vi "Thread@Suspend__Parameter.vi"(1 "ParamterIn":string) -> (0 "ParamterOut":string)   [LabVIEW 2020]
panel:
  in  "Logic":string(combo)
  in  "Thread":string(combo)="1"
  in  "Confirm":bool
  # "Thread@Suspend $ThreadNo (, $Logic)"
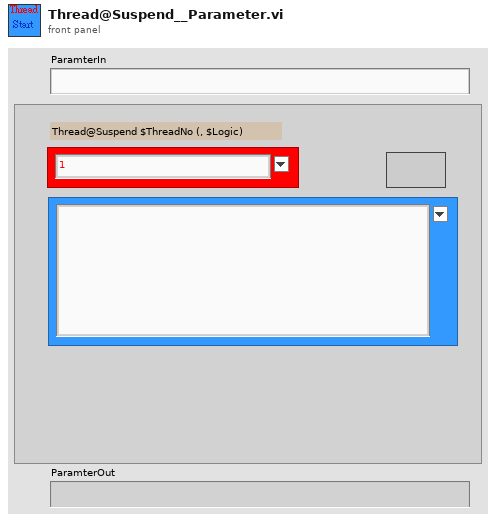
[diagram p1: front panel]
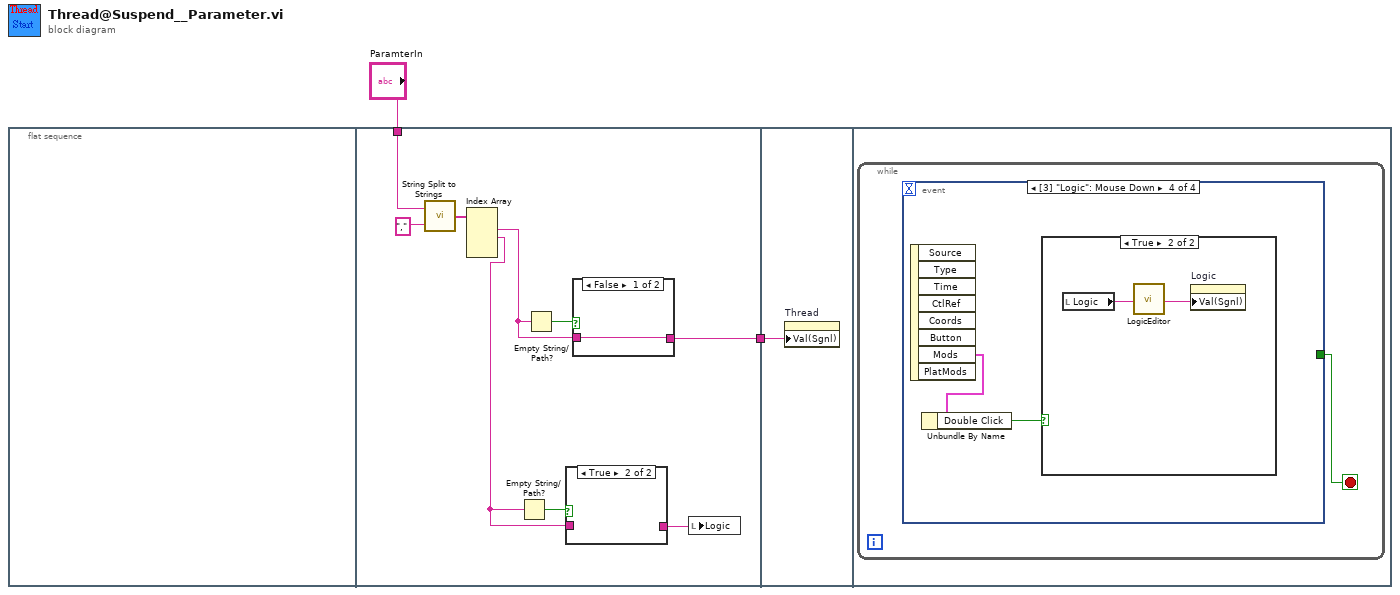
[diagram p0: block diagram]
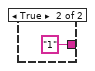
[diagram p3: hidden frame]
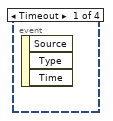
[diagram p4: hidden frame]
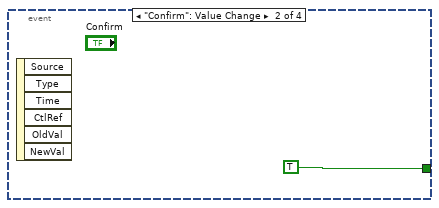
[diagram p5: hidden frame]
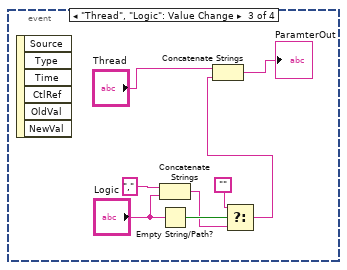
[diagram p6: hidden frame]
diagram:
  n1 = flat-sequence {
    tunnel: "ParamterIn" -> [w9]
    tunnel: [w3] -> w1
    tunnel: w1 -> [w15]
    frame #0 {
    }
    frame #1 {
      n2 = call "String Split to Strings.vi"("search string/char (-)"=",", "String"=w9) -> ("Array"=w11:string[])
      n3 = Index Array(array=w11) -> (element #1=w5:string, element #2=w4:string)  [unwired: 4 in, 2 out]
      n4 = Empty String/Path?(string/path=w4) -> (empty?=w7:bool)
      n5 = Empty String/Path?(string/path=w5) -> (empty?=w8:bool)
      n6 = case shown="True" w7 {
        tunnel: w4 -> [w12 _]
        tunnel: [w12 _] -> w6
        frame False {
        }
        frame True {
        }
      }
      n7 = case shown="False" w8 {
        tunnel: w5 -> [w13 _]
        tunnel: [w13 "1"] -> w3
        frame False {
        }
        frame True {
        }
      }
      n8 = local write "Logic"(w6) -> ()
    }
    frame #2 {
      n9 = property on="Thread" class="CmbBox"("Val(Sgnl)"=w15) -> ()  [unwired: 2 in, 2 out]
    }
    frame #3 {
      n10 = while {
        stop <- w16 stop-if-true
        n11 = event shown="[3] \"Logic\": Mouse Down" {
          selector: _ -> [_ _ _ _]
          dyn-events: _ -> [_ _ _ _]
          timeout: _ -> [_ _ _ _]
          tunnel: [_ TRUE _ _] -> w16
          event Timeout {
            n12 = event-data() -> ()  [unwired: 1 in, 3 out]
          }
          event "Confirm": Value Change {
            n13 = event-data() -> ()  [unwired: 1 in, 6 out]
          }
          event "Thread", "Logic": Value Change {
            n14 = event-data() -> ()  [unwired: 1 in, 6 out]
            n15 = Concatenate Strings("," ("string"), "Logic") -> (w21:string)
            n16 = Empty String/Path?(string/path="Logic") -> (empty?=w24:bool)
            n17 = Select(t="", s=w24, f=w21) -> (s? t:f=w20:string)
            n18 = Concatenate Strings("Thread", w20) -> (→"ParamterOut":string)
          }
          event "Logic": Mouse Down {
            n19 = event-data() -> ("Mods"=w27:cluster{"Double Click":bool, "Menu Key":bool})  [unwired: 1 in, 7 out]
            n20 = Unbundle By Name(w27) -> ("Double Click"=w26:bool)
            n21 = case shown="True" w26 {
              frame False {
              }
              frame True {
                n22 = local read "Logic"() -> (w29:string)
                n23 = call "LogicEditor.vi"("Logic Express"=w29) -> ("LogicExpressOut"=w28:string)
                n24 = property on="Logic" class="CmbBox"("Val(Sgnl)"=w28) -> ()  [unwired: 2 in, 2 out]
              }
            }
          }
        }
      }
    }
  }
